vi "CRHKitToExcel.vi"() -> ()   [LabVIEW 2012]
uses:
  <vilib>/addons/database/Auxilliary.llb/DB Tools Cursor Type.ctl
  <vilib>/Utility/NIReport.llb/NI_report.lvclass
  <vilib>/addons/database/Connection.llb/DB Tools Open Connec (Path).vi
  <vilib>/addons/database/Connection.llb/Conn Execute.vi
  <vilib>/addons/database/Recordset.llb/Rec Fetch Recordset Data (R).vi
  <vilib>/addons/database/Recordset.llb/Rec Destroy - Connection.vi
  <vilib>/addons/database/_DB Variant To Data/Database Variant To Data.xnode
  <vilib>/addons/database/NI_Database_API.lvlib
  <vilib>/Utility/NIReport.llb/Excel/NI_Excel.lvclass
  <vilib>/Utility/SMTP/NI_SMTPEmail.lvlib
panel:
  out "concatenated string":string
  out "error out 2":errorcluster
  in  "MIME content-type (application/octet-stream)":string="application/octet-stream"
  out "error out":errorcluster
  out "error out 3":errorcluster
  in  "?":cluster{"start row":i32, "start column":i32}
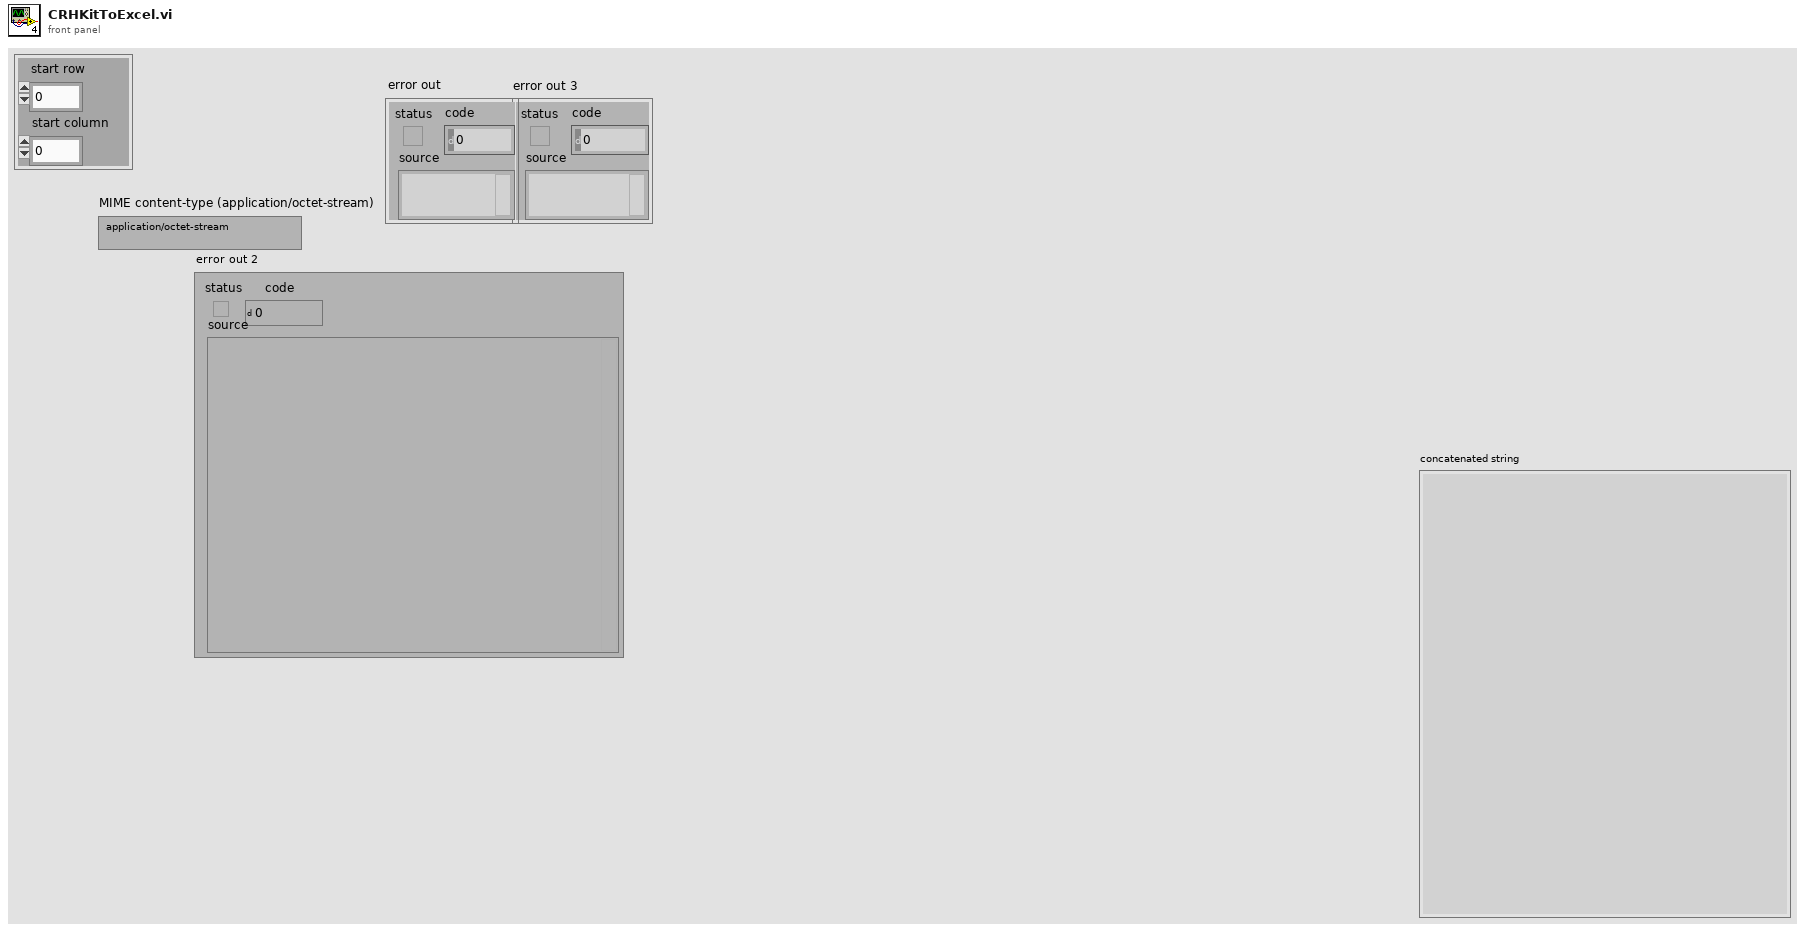
[diagram p1: front panel]
types:
  T1 = enum16{"Standard Report", "HTML", "Word", "Excel"}
  T2 = typedef "NI_Database_API.lvlib/Conn ObjectReference.ctl" = refnum<k1>
  T3 = typedef "NI_Database_API.lvlib/DB Tools Cursor Type.ctl" = enum16{"forward-only", "keyset", "dynamic", "static"}
  T4 = typedef "NI_Database_API.lvlib/Rec ObjectReference.ctl" = refnum<k1>
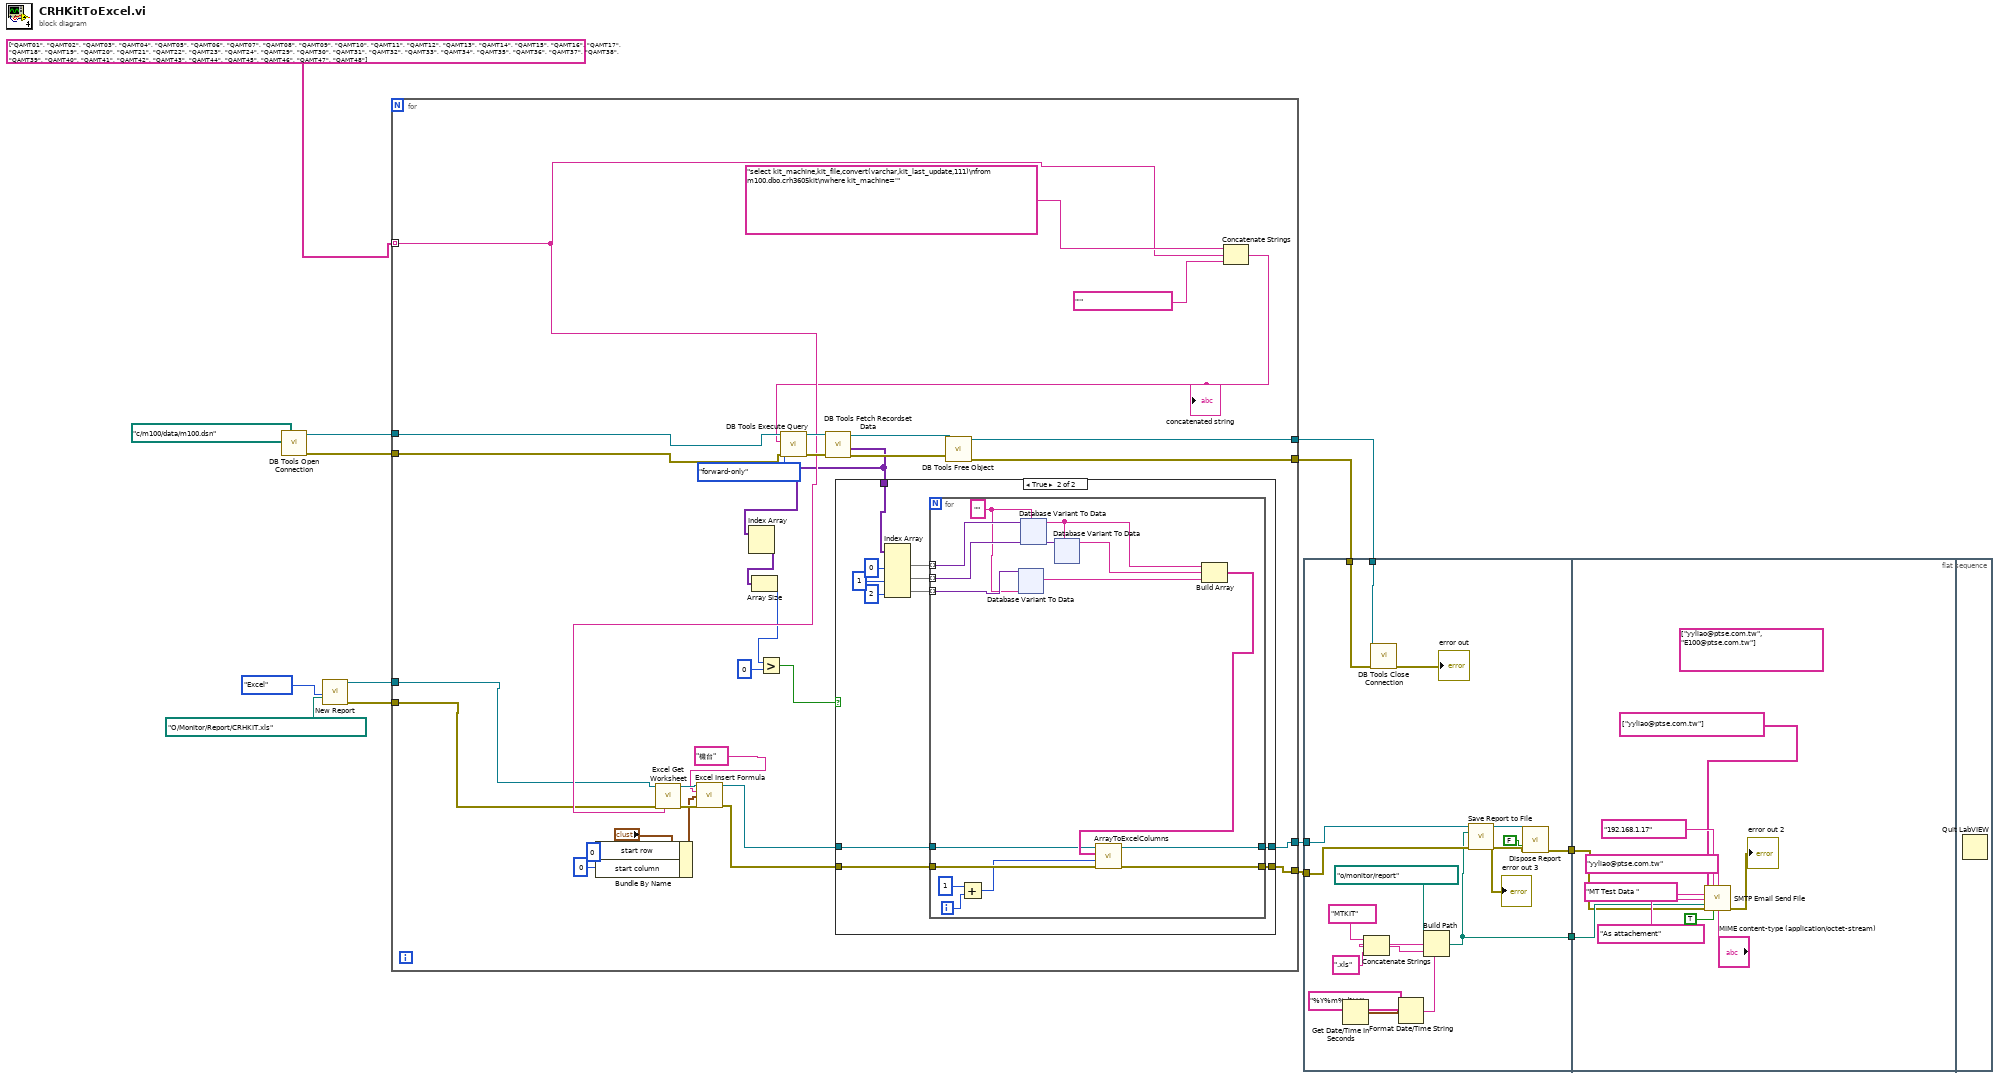
[diagram p0: block diagram]
diagram:
  n1 = call-poly <vilib>:"DB Tools Open Connection.vi"("connection information"=path "c:/m100/data/m100.dsn") -> ("error out"=w4:errorcluster, "connection reference"=w5:T2)  [unwired: 7 in]
  n2 = call <vilib>:"New Report.vi"("report type"=T1."Excel" ("Report Type"), "template (empty)"=path "O:/Monitor/Report/CRHKIT.xls") -> ("report out"=w8:refnum<class "NI_report.lvclass">, "error out"=w7:errorcluster)  [unwired: 12 in]
  n3 = for {
    tunnel: [w30] -> w12
    tunnel: [w29] -> w11
    tunnel: string[] ["QAMT01", "QAMT02", "QAMT03", "QAMT04", "QAMT05", "QAMT06", "QAMT07", "QAMT08", "QAMT09", "QAMT10", "QAMT11", "QAMT12", "QAMT13", "QAMT14", "QAMT15", "QAMT16", "QAMT17", "QAMT18", "QAMT19", "QAMT20", "QAMT21", "QAMT22", "QAMT23", "QAMT24", "QAMT29", "QAMT30", "QAMT31", "QAMT32", "QAMT33", "QAMT34", "QAMT35", "QAMT36", "QAMT37", "QAMT38", "QAMT39", "QAMT40", "QAMT41", "QAMT42", "QAMT43", "QAMT44", "QAMT45", "QAMT46", "QAMT47", "QAMT48"] ("Array") -> [w28] mode=indexing
    tunnel: w8 -> [w27]
    tunnel: w7 -> [w26]
    tunnel: w5 -> [w25]
    tunnel: w4 -> [w24]
    tunnel: [w23] -> w2
    tunnel: [w22] -> w1
    n4 = Bundle By Name(cluster="?", "start row"=0, "start column"=0) -> (w33:cluster{"start row":i32, "start column":i32})
    n5 = call <vilib>:"Excel Get Worksheet.vi"("report in"=w27, "error in (no error)"=w26, "name (\"\")"=w28) -> ("report out"=w38:refnum<class "NI_report.lvclass">, "error out"=w37:errorcluster)  [unwired: 11 in]
    n6 = call <vilib>:"Excel Insert Formula.vi"("report in"=w38, "formula"="機台", "start (0, 0)"=w33, "error in (no error)"=w37) -> ("report out"=w32:refnum<class "NI_report.lvclass">, "error out"=w31:errorcluster)  [unwired: 10 in]
    n7 = Concatenate Strings("select kit_machine,kit_file,convert(varchar,kit_last_update,111)\nfrom m100.dbo.crh3605kit\nwhere kit_machine='" ("SQL query"), w28, "'" ("SQL query")) -> (w16:string)
    "concatenated string" <- w16
    n8 = call-poly <vilib>:"DB Tools Execute Query.vi"("error in (no error)"=w24, "cursor type"=DB_Tools_Cursor_Type."forward-only", "SQL query"=w16, "connection reference"=w25) -> ("error out"=w45:errorcluster, "recordset reference"=w44:T4)  [unwired: 4 in]
    n9 = call-poly <vilib>:"DB Tools Fetch Recordset Data.vi"("error in (no error)"=w45, "recordset reference"=w44) -> ("error out"=w42:errorcluster, "recordset data"=w21:variant[][], "recordset reference out"=w43:T4)  [unwired: 3 in]
    n10 = Index Array(array=w21) -> (element=w20:variant[])  [unwired: 2 in]
    n11 = Array Size(array=w20) -> (size(s)=w19:i32)
    n12 = Greater?(x=w19, y=0) -> (0:w17:bool)
    n13 = case shown="True" w17 {
      tunnel: w21 -> [_ w58]
      tunnel: w32 -> [w47 w51]
      tunnel: w31 -> [w46 w50]
      tunnel: [w47 w49] -> w30
      tunnel: [w46 w48] -> w29
      frame False {
      }
      frame True {
        n14 = Index Array(array=w58, index (col) #1=0 ("disabled index (col)"), index (col) #2=1 ("index (col)"), index (col) #3=2 ("index (col)")) -> (element #1=w55:variant[], element #2=w54:variant[], element #3=w53:variant[])  [unwired: 3 in]
        n15 = for {
          tunnel: w55 -> [w73] mode=indexing
          tunnel: w54 -> [w72] mode=indexing
          tunnel: w53 -> [w71] mode=indexing
          tunnel: w51 -> [w66]
          tunnel: w50 -> [w65]
          tunnel: [w61] -> w49
          tunnel: [w60] -> w48
          i -> [w64]
          w59 = ""
          n16 = Add(x=1, y=w64) -> (x+y=w62:i32)
          n17 = xnode "Database Variant To Data"("database variant"=w71, "type"=w59) -> ("data"=w68:string)  [unwired: 1 in, 1 out]
          n18 = xnode "Database Variant To Data"("database variant"=w73, "type"=w59) -> ("data"=w69:string)  [unwired: 1 in, 1 out]
          n19 = xnode "Database Variant To Data"("database variant"=w72, "type"=w69) -> ("data"=w70:string)  [unwired: 1 in, 1 out]
          n20 = Build Array(w69, w70, w68) -> (w67:string[])
          n21 = call "ArrayToExcelColumns.vi"("error in (no error)"=w65, "start row"=w62, "ArrayData"=w67, "report in"=w66) -> ("error in (no error) 2"=w60:errorcluster, "report in 2"=w61:refnum<class "NI_report.lvclass">)  [unwired: 6 in]
        }
      }
    }
    n22 = call-poly <vilib>:"DB Tools Free Object.vi"("error in (no error)"=w42, "recordset reference"=w43) -> ("error out"=w22:errorcluster, "connection reference"=w23:T2)  [unwired: 8 in]
  }
  n23 = flat-sequence {
    tunnel: w12 -> [w182]
    tunnel: w11 -> [w181]
    tunnel: w2 -> [w172]
    tunnel: w1 -> [w171]
    tunnel: [w175] -> w14
    tunnel: [w174] -> w13
    tunnel: w14 -> [w188]
    tunnel: w13 -> [w189]
    frame #0 {
      n24 = Get Date/Time In Seconds() -> (seconds since 1Jan1904=w178:timestamp)
      n25 = call <vilib>:"DB Tools Close Connection.vi"("error in (no error)"=w171, "connection reference"=w172) -> ("error out"=→"error out":errorcluster)  [unwired: 5 in]
      n26 = Format Date/Time String(time format string (%c)="%Y%m%d%H", seconds (now)=w178) -> (date/time string=w176:string)  [unwired: 1 in]
      n27 = Concatenate Strings("MTKIT" ("string"), w176, ".xls" ("string")) -> (w183:string)
      n28 = Build Path(base path=path "o:/monitor/report", name or relative path=w183) -> (appended path=w174:path)
      n29 = call-dynamic "Save Report to File.vi"("report in"=w182, "report file path"=w174, "error in (no error)"=w181) -> ("report out"=w185:refnum<class "NI_report.lvclass">, "error out"=w184:errorcluster)  [unwired: 11 in]
      "error out 3" <- w184
      n30 = call-dynamic "Dispose Report.vi"("report in"=w185, "save changes? (F)"=FALSE, "error in (no error)"=w184) -> ("error out"=w175:errorcluster)  [unwired: 12 in]
    }
    frame #1 {
      (unwired) string[] ["yyliao@ptse.com.tw", "E100@ptse.com.tw"] ("recipients")
      n31 = call <vilib>:"SMTP Email Send File.vi"("recipients"=string[] ["yyliao@ptse.com.tw"], "mail server"="192.168.1.17", "return address"="yyliao@ptse.com.tw", "subject ([No Subject])"="MT Test Data ", "message"="As attachement", "file path"=w189, "error in (no error)"=w188, "binary? (F)"=TRUE, "MIME content-type (application/octet-stream)"="MIME content-type (application/octet-stream)") -> ("error out"=→"error out 2":errorcluster)  [unwired: 5 in, 1 out]
    }
    frame #2 {
      n32 = Quit LabVIEW() -> ()  [unwired: 1 in]
    }
  }
